vi "VI2.vi"   [LabVIEW 2012]
uses:
  <vilib>/rvi/interface/nirviOpenFPGA/nirviOpenFPGA.xnode
  ModuleTest1_FPGATarget_VI1_0LoCP9tHAE0.lvbitx
  <vilib>/FPGAPlugInAG/cRIO-9081/niLvFpga_Open_cRIO-9081.vi
  <vilib>/rvi/interface/common/dynamic/niFpgaDynamicAddResources.vi
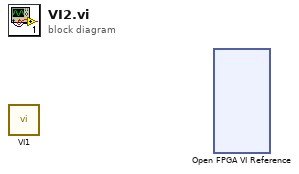
[diagram p0: block diagram]
diagram:
  n1 = call "VI1.vi"() -> ()  [unwired: 1 out]
  n2 = xnode "Open FPGA VI Reference"() -> ()  [unwired: 2 in, 2 out]
